vi "DestroyBroadcastEvents.vi"(8 "error in (no error)":errorcluster) -> (0 "error out":errorcluster)   [LabVIEW 2018, in "MyPlugins.lvlib"]
doc: "Closes the user events generated that describe which broadcasts can be sent from the module."
uses:
  MyPlugins.lvlib
  PluginsShared/clBroadcastEvents.ctl
  PluginsShared/clEventType.ctl
  PluginsShared/PluginsShared.lvlib
panel:
  out "clBroadcastEvents":T1
  # "If you want to add other Broadcast Events, open this typedef, copy an existing event and rename it to your event name.\n\nNext create an \"arg\" typedef for the  data and put it into PublicAPI/Arguments/Broadcasts\n\nAfter that, you will need to create a new roadcast vi in Protected/Broadcast.  Look at DidInit.vi or the reportError.vi as examples."
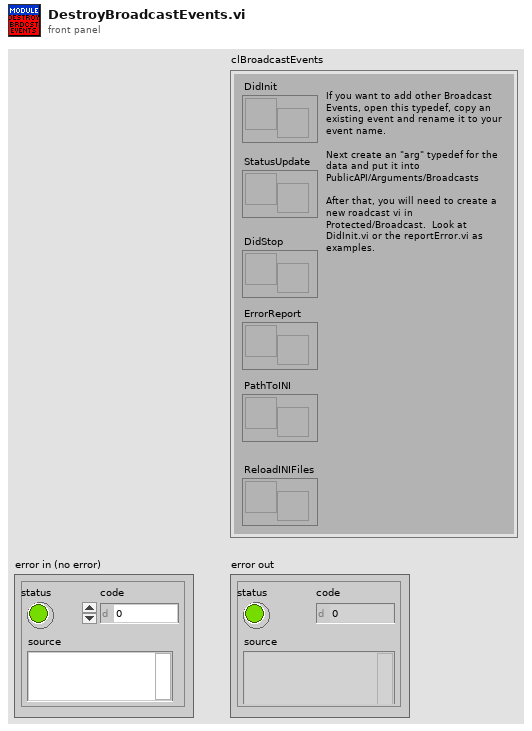
[diagram p1: front panel]
types:
  T1 = typedef "PluginsShared.lvlib/clBroadcastEvents.ctl" = cluster{"DidInit":refnum<user-event>, "StatusUpdate":refnum<user-event>, "ErrorReport":refnum<user-event>, "DidStop":refnum<user-event>, "PathToINI":refnum<user-event>, "ReloadINIFiles":refnum<user-event>}
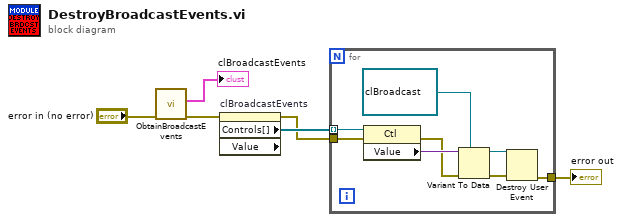
[diagram p0: block diagram]
diagram:
  n1 = call "ObtainBroadcastEvents.vi"("error in (no error)"="error in (no error)") -> ("error out"=w2:errorcluster, "clBroadcastEvents"=→"clBroadcastEvents":T1)  [unwired: 9 in]
  n2 = property on="clBroadcastEvents" class="Clust (strict)" props=["Controls[]", "Value"](error in=w2) -> (error out=w1:errorcluster, "Controls[]"=w5:refnum<vi>[])  [unwired: 1 in, 2 out]
  n3 = for {
    tunnel: w5 -> [w14] mode=indexing
    tunnel: w1 -> [w8]
    tunnel: [w11] -> w6
    n4 = property class="Ctl"(reference=w14, error in=w8) -> (error out=w7:errorcluster, "Value"=w13:variant)  [unwired: 1 out]
    n5 = Variant To Data(error in=w7, type=refnum<user-event> refnum ("DidInit"), Variant=w13) -> (data=w10:refnum<user-event>, error out=w12:errorcluster)
    n6 = Destroy User Event(user event=w10, error in=w12) -> (error out=w11:errorcluster)
  }
  "error out" <- w6
